vi "convert To Voltage.vi"(9 "value":u16, 10 "adcCh":u32, 11 "instance":i32) -> (3 "function return":dbl)   [LabVIEW 2022 SP3, in "SADI_FW3.lvlib"]
doc: "SADI_API_Wrapper double convertToVoltage(int instance, unsigned int adcCh, uint16_t value);"
uses:
  SADI_FW3.lvlib
  SADI_FW3.dll
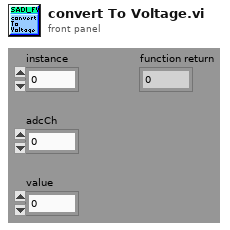
[diagram p1: front panel]
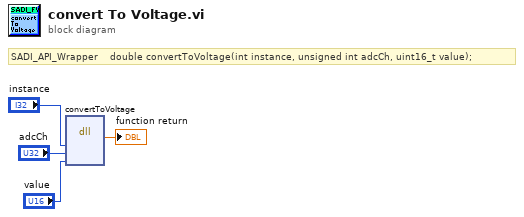
[diagram p0: block diagram]
diagram:
  # "SADI_API_Wrapper    double convertToVoltage(int instance, unsigned int adcCh, uint16_t value);"
  n1 = dll-call lib="C:/Users/scer/OneDrive - University of Florida/eml4314c/eml4314SP23/resources/release_2_3_23/LV/LVLib/SADI_FW3.*" fn="convertToVoltage"("instance"="instance", "adcCh"="adcCh", "value"="value") -> (→"function return":dbl)  [unwired: 6 in, 2 out]
